vi "Send Set Virtual Instr Configuration.vi"(7 "Message Priority (Normal)":T1=enum."Normal", 8 "error in (no error)":errorcluster, 10 "Virt Instr CFG":string, 11 "Message Enqueuer":refnum<class "Message Enqueuer.lvclass">) -> (0 "error out":errorcluster, 3 "Message Enqueuer out":refnum<class "Message Enqueuer.lvclass">)   [LabVIEW 2023, in "IConfiguration UI Actor.lvlib" / "Set Virtual Instr Configuration Msg.lvclass"]
doc: "This VI sends the message to an actor."
uses:
  Set Virtual Instr Configuration Msg.lvclass
  Set Virtual Instr Configuration Msg.lvclass/Set Virtual Instr Configuration Msg.ctl
  <vilib>/ActorFramework/Message Enqueuer/Message Enqueuer.lvclass
  C:/Program Files (x86)/National Instruments/LabVIEW 2023/vi.lib/ActorFramework/Message/Message.lvclass
  E:/git/HAL/Configurator/IConfiguration UI Actor/IConfiguration UI Actor Messages/Set Virtual Instr Configuration Msg/Set Virtual Instr Configuration Msg.lvclass
  <vilib>/ActorFramework/Message Enqueuer/Message Priority.ctl
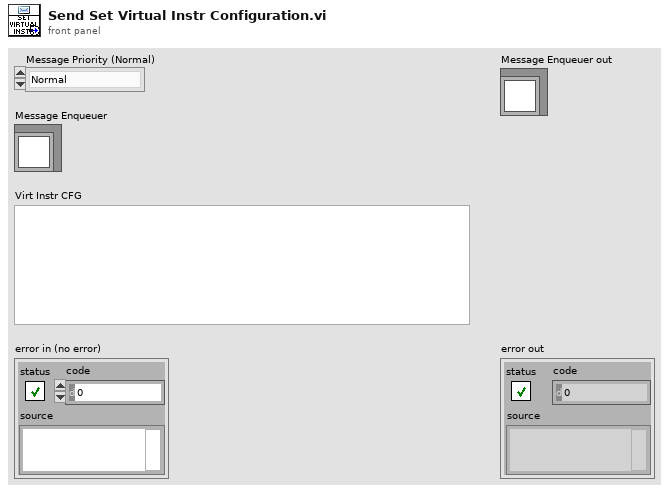
[diagram p1: front panel]
types:
  T1 = typedef "Actor Framework.lvlib/Message Enqueuer.lvclass/Message Priority.ctl" = enum16{"Low", "Normal", "High"}
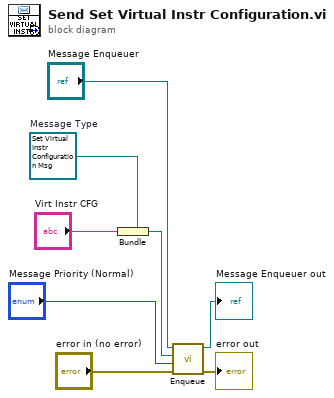
[diagram p0: block diagram]
diagram:
  w5 = refnum<class "Set Virtual Instr Configuration Msg.lvclass"> refnum  # Message Type
  n1 = Bundle(cluster=w5, "Virt Instr CFG") -> (w4:refnum<class "Set Virtual Instr Configuration Msg.lvclass">)
  n2 = call <vilib>:"Enqueue.vi"("error in (no error)"="error in (no error)", "Message Priority (Normal)"="Message Priority (Normal)", "Message"=w4, "Message Enqueuer in"="Message Enqueuer") -> ("error out"=→"error out":errorcluster, "Message Enqueuer in"=→"Message Enqueuer out":refnum<class "Message Enqueuer.lvclass">)  [unwired: 6 in]
